vi "color_sensor_vibhu.vi"() -> ()   [LabVIEW 2022 SP3]
uses:
  <vilib>/DAQmx/write.llb/DAQmx Write (Digital Bool 1Line 1Point).vi
  <vilib>/DAQmx/create/channels.llb/DAQmx Create Channel (DO-Digital Output).vi
  <vilib>/DAQmx/miscellaneous.llb/DAQmx Fill In Error Info.vi
  <vilib>/Instr/_visa.llb/VISA Configure Serial Port (Instr).vi
panel:
  out "read buffer 2":string
  in  "stop":bool
  in  "VISA resource name 2":refnum<visa-resource-name>
  out "Numeric":i32
  out "red":bool
  out "blue":bool
  out "green":bool
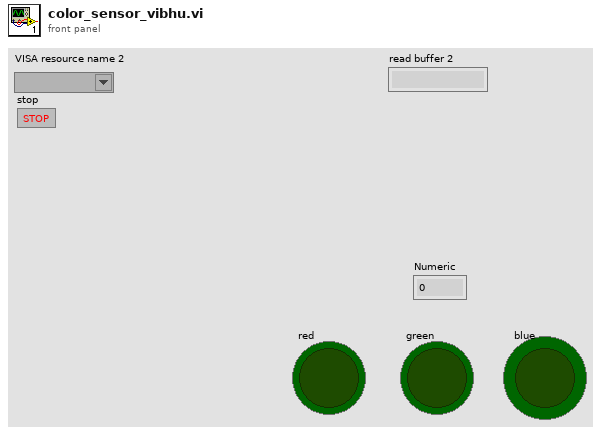
[diagram p1: front panel]
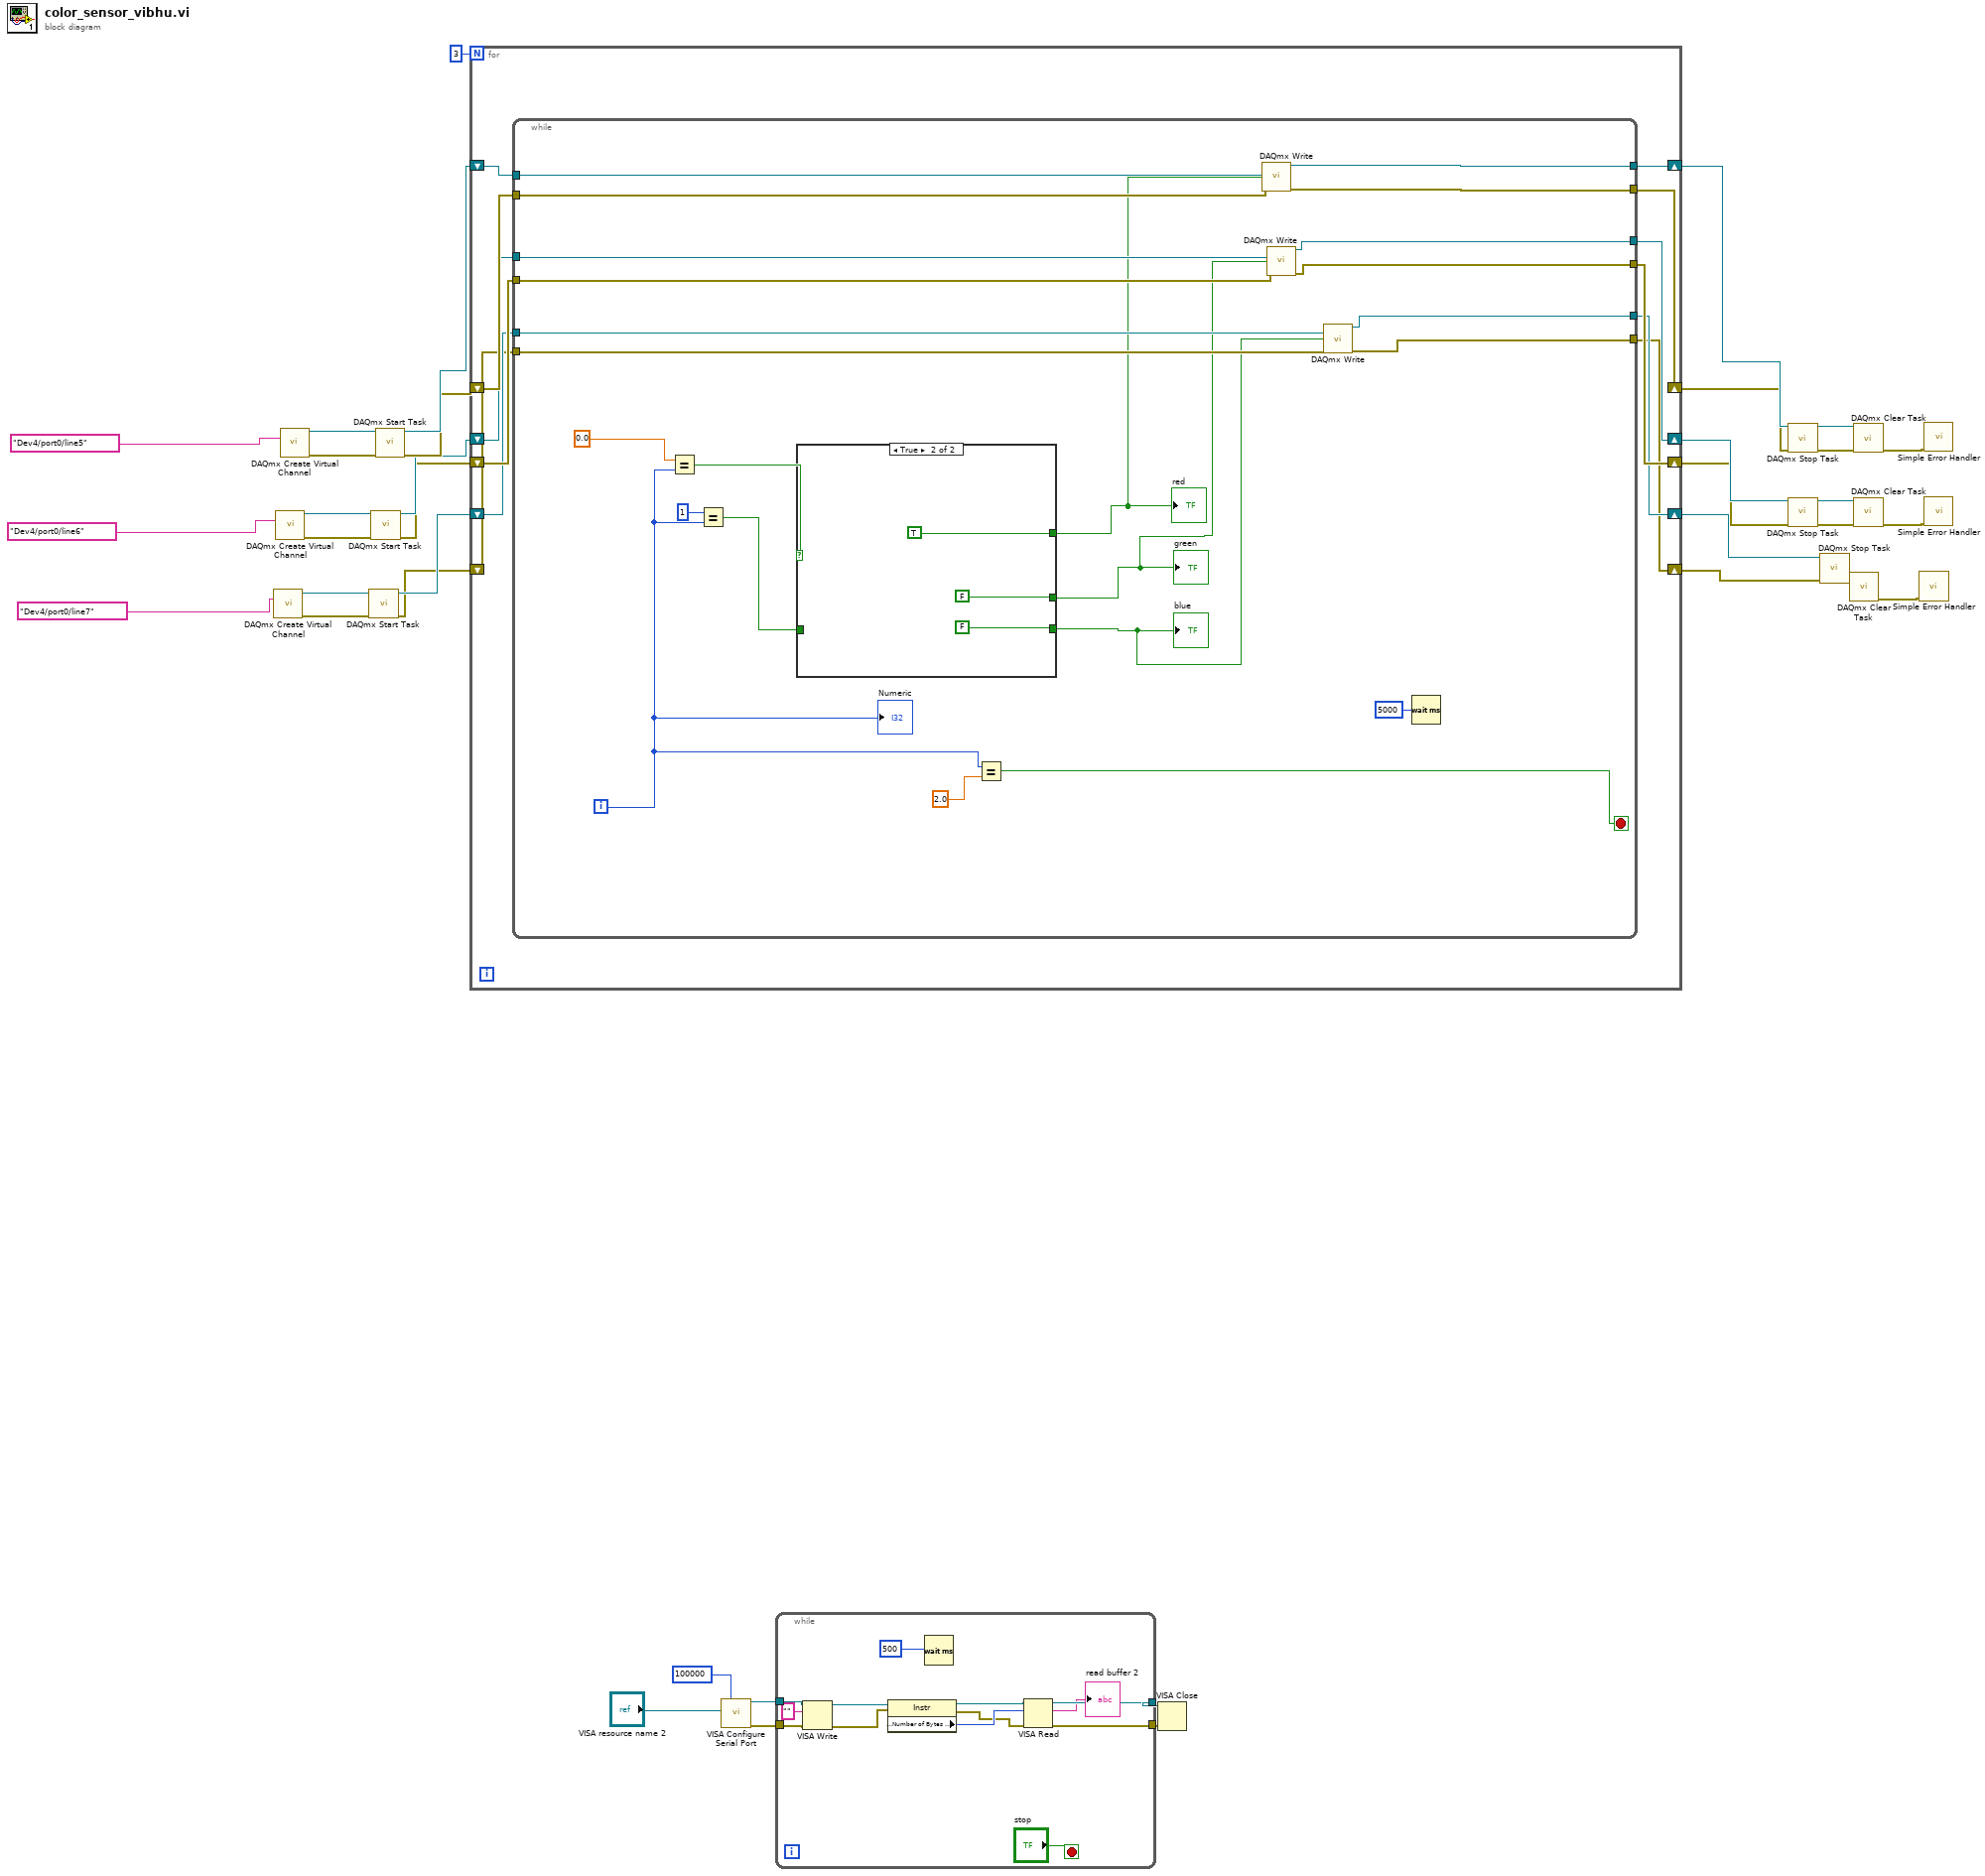
[diagram p0: block diagram]
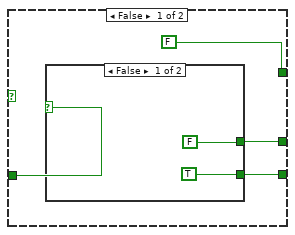
[diagram p2: hidden frame]
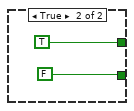
[diagram p3: hidden frame]
diagram:
  n1 = call-poly <vilib>:"DAQmx Create Virtual Channel.vi"("lines"=tag "Dev4/port0/line7" ("Blue Channel")) -> ("task out"=w26:refnum<k21>, "error out"=w27:errorcluster)  [unwired: 13 in]
  n2 = call-poly <vilib>:"DAQmx Create Virtual Channel.vi"("lines"=tag "Dev4/port0/line6" ("Green Channel")) -> ("task out"=w31:refnum<k21>, "error out"=w32:errorcluster)  [unwired: 13 in]
  n3 = call-poly <vilib>:"DAQmx Create Virtual Channel.vi"("lines"=tag "Dev4/port0/line5" ("Red Channel")) -> ("task out"=w36:refnum<k21>, "error out"=w37:errorcluster)  [unwired: 13 in]
  n4 = call <vilib>:"DAQmx Start Task.vi"("task/channels in"=w26, "error in"=w27) -> ("task out"=w15:refnum<k21>, "error out"=w14:errorcluster)  [unwired: 12 in]
  n5 = call <vilib>:"DAQmx Start Task.vi"("task/channels in"=w31, "error in"=w32) -> ("task out"=w17:refnum<k21>, "error out"=w16:errorcluster)  [unwired: 12 in]
  n6 = call <vilib>:"DAQmx Start Task.vi"("task/channels in"=w36, "error in"=w37) -> ("task out"=w19:refnum<k21>, "error out"=w18:errorcluster)  [unwired: 12 in]
  n7 = for {
    N: 3 -> [_]
    shift-right: [w43] -> w13
    shift-left: w19 -> [w49]
    shift-right: [w42] -> w12
    shift-left: w18 -> [w48]
    shift-right: [w41] -> w11
    shift-left: w17 -> [w47]
    shift-right: [w40] -> w10
    shift-left: w16 -> [w46]
    shift-right: [w39] -> w9
    shift-left: w15 -> [w45]
    shift-right: [w38] -> w8
    shift-left: w14 -> [w44]
    n8 = while {
      tunnel: w49 -> [w64]
      tunnel: w48 -> [w63]
      tunnel: [w62] -> w43
      tunnel: [w61] -> w42
      tunnel: w47 -> [w60]
      tunnel: w46 -> [w59]
      tunnel: [w58] -> w41
      tunnel: [w57] -> w40
      tunnel: w45 -> [w56]
      tunnel: w44 -> [w55]
      tunnel: [w54] -> w39
      tunnel: [w53] -> w38
      i -> [w66]
      stop <- w71 stop-if-true
      n9 = Equal?(x=0.0, y=w66) -> (x = y?=w68:bool)
      n10 = Equal?(x=1, y=w66) -> (x = y?=w67:bool)
      n11 = case shown="True" w68 {
        tunnel: [FALSE TRUE] -> w52
        tunnel: w67 -> [w76 _]
        tunnel: [w74 FALSE] -> w51
        tunnel: [w73 FALSE] -> w50
        frame False {
          n12 = case shown="False" w76 {
            tunnel: [FALSE TRUE] -> w74
            tunnel: [TRUE FALSE] -> w73
            frame False {
            }
            frame True {
            }
          }
        }
        frame True {
        }
      }
      "red" <- w52
      "blue" <- w50
      "green" <- w51
      n13 = Equal?(x=w66, y=2.0) -> (x = y?=w71:bool)
      n14 = call-poly <vilib>:"DAQmx Write.vi"("task/channels in"=w64, "data"=w52, "error in"=w63) -> ("task out"=w62:refnum<k21>, "error out"=w61:errorcluster)  [unwired: 10 in, 1 out]
      n15 = call-poly <vilib>:"DAQmx Write.vi"("task/channels in"=w60, "data"=w51, "error in"=w59) -> ("task out"=w58:refnum<k21>, "error out"=w57:errorcluster)  [unwired: 10 in, 1 out]
      n16 = call-poly <vilib>:"DAQmx Write.vi"("task/channels in"=w56, "data"=w50, "error in"=w55) -> ("task out"=w54:refnum<k21>, "error out"=w53:errorcluster)  [unwired: 10 in, 1 out]
      n17 = Wait (ms)(milliseconds to wait=u32 5000) -> ()  [unwired: 1 out]
      "Numeric" <- w66
    }
  }
  n18 = call-poly "VISA Configure Serial Port"("VISA resource name"="VISA resource name 2", "timeout (10sec)"=u32 100000) -> ("VISA resource name out"=w4:refnum<visa-resource-name>, "error out"=w3:errorcluster)  [unwired: 12 in]
  n19 = while {
    tunnel: w4 -> [w95]
    tunnel: w3 -> [w94]
    tunnel: [w88] -> w2
    tunnel: [w87] -> w1
    stop <- "stop" stop-if-true
    n20 = VISA Write(VISA resource name=w95, write buffer="", error in (no error)=w94) -> (VISA resource name out=w93:refnum<visa-resource-name>, error out=w92:errorcluster)  [unwired: 1 out]
    n21 = property class="Instr"(reference=w93, error in=w92) -> (reference out=w90:refnum<visa-resource-name>, error out=w89:errorcluster, "Serial Settings:Number of Bytes at Serial Port"=w91:u32)
    n22 = Wait (ms)(milliseconds to wait=u32 500 ("millisecond timer value")) -> ()  [unwired: 1 out]
    n23 = VISA Read(VISA resource name=w90, byte count=w91, error in (no error)=w89) -> (VISA resource name out=w88:refnum<visa-resource-name>, read buffer=→"read buffer 2":string, error out=w87:errorcluster)  [unwired: 1 out]
  }
  n24 = VISA Close(VISA resource name=w2, error in (no error)=w1) -> ()  [unwired: 1 out]
  n25 = call <vilib>:"DAQmx Stop Task.vi"("task/channels in"=w13, "error in"=w12) -> ("task out"=w35:refnum<k21>, "error out"=w34:errorcluster)  [unwired: 12 in]
  n26 = call <vilib>:"DAQmx Stop Task.vi"("task/channels in"=w11, "error in"=w10) -> ("task out"=w30:refnum<k21>, "error out"=w29:errorcluster)  [unwired: 12 in]
  n27 = call <vilib>:"DAQmx Stop Task.vi"("task/channels in"=w9, "error in"=w8) -> ("task out"=w25:refnum<k21>, "error out"=w24:errorcluster)  [unwired: 12 in]
  n28 = call <vilib>:"DAQmx Clear Task.vi"("task in"=w25, "error in"=w24) -> ("error out"=w23:errorcluster)  [unwired: 13 in]
  n29 = call <vilib>:"DAQmx Clear Task.vi"("task in"=w35, "error in"=w34) -> ("error out"=w33:errorcluster)  [unwired: 13 in]
  n30 = call <vilib>:"DAQmx Clear Task.vi"("task in"=w30, "error in"=w29) -> ("error out"=w28:errorcluster)  [unwired: 13 in]
  n31 = call <vilib>:"Simple Error Handler.vi"("error in (no error)"=w23) -> ()  [unwired: 4 in, 5 out]
  n32 = call <vilib>:"Simple Error Handler.vi"("error in (no error)"=w33) -> ()  [unwired: 4 in, 5 out]
  n33 = call <vilib>:"Simple Error Handler.vi"("error in (no error)"=w28) -> ()  [unwired: 4 in, 5 out]
